vi "ReadPath.vi"(8 "error in (no error)":errorcluster, 11 "AI_Snake in":refnum<class "AI_Snake.lvclass">) -> (0 "error out":errorcluster, 3 "AI_Snake out":refnum<class "AI_Snake.lvclass">)   [LabVIEW 2019, in "RT_Game.lvlib" / "AI_Snake.lvclass"]
uses:
  AI_Snake.lvclass
  C:/Users/FreshBob/Dropbox/VIs/myRIO_GameConsole/RT/RT_Game/Snake/Snake.lvclass
  Engine/Coordinate.ctl
  AI_Snake.lvclass/AI_Snake.ctl
  Snake/Snake.lvclass/Snake.ctl
  Snake/Read Length.vi
  Snake/Write Position (Tiles).vi
  Engine/Engine.lvclass
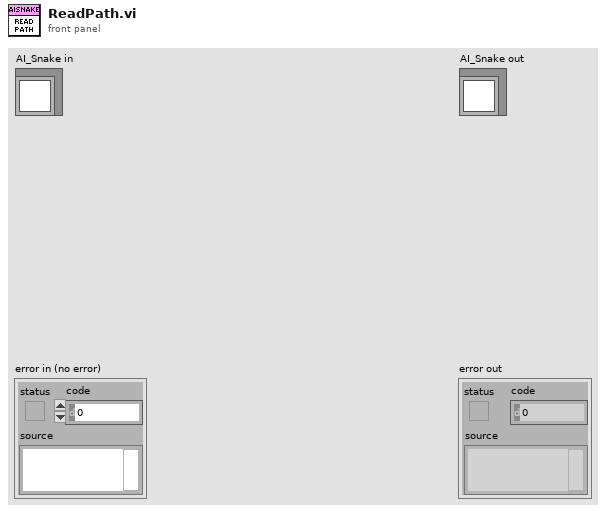
[diagram p1: front panel]
types:
  T1 = typedef "RT_Game.lvlib/Engine.lvclass/Coordinate.ctl" = cluster{"x":dbl, "y":dbl}
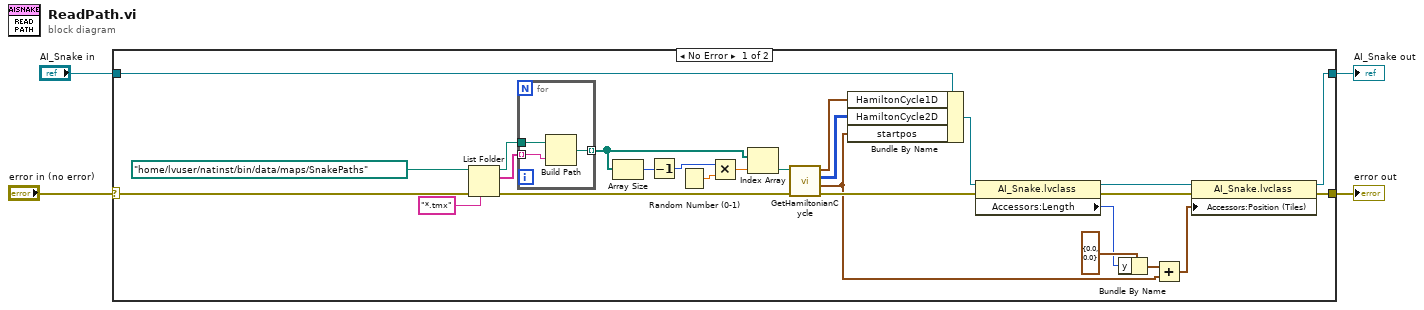
[diagram p0: block diagram]
diagram:
  n1 = case shown="No Error" "error in (no error)" {
    selector: "error in (no error)" -> [w24 w35]
    tunnel: [w23 w35] -> w3
    tunnel: [w21 w34] -> w1
    tunnel: "AI_Snake in" -> [w22 w34]
    frame No Error {
      n2 = List Folder(path=path "/home/lvuser/natinst/bin/data/maps/SnakePaths", pattern="*.tmx", error in=w24) -> (path out=w11:path, filenames=w12:string[], error out=w15:errorcluster)  [unwired: 1 in, 1 out]
      n3 = for {
        tunnel: w12 -> [w33] mode=indexing
        tunnel: w11 -> [w32]
        tunnel: [w31] -> w10 mode=indexing
        n4 = Build Path(base path=w32, name or relative path=w33) -> (appended path=w31:path)
      }
      n5 = Array Size(array=w10) -> (size(s)=w9:i32)
      n6 = Decrement(x=w9) -> (x-1=w7:i32)
      n7 = Random Number (0-1)() -> (number: 0 to 1=w8:dbl)
      n8 = Multiply(x=w7, y=w8) -> (x*y=w6:dbl)
      n9 = Index Array(array=w10, index=w6) -> (element=w5:path)
      n10 = call "GetHamiltonianCycle.vi"("error in (no error)"=w15, "path to tmx-file (created with Tiles2D)"=w5) -> ("error out"=w28:errorcluster, "startpos"=w20:cluster{i32, i32}, "Hamilton2D"=w25:u32[][], "Hamilton1D"=w26:cluster{i32, i32}[])  [unwired: 6 in]
      n11 = Bundle By Name(cluster=w22, "HamiltonCycle1D"=w26, "HamiltonCycle2D"=w25, "startpos"=w20) -> (w27:refnum<class "AI_Snake.lvclass">)
      n12 = property class="AI_Snake.lvclass"(reference=w27, error in=w28) -> (reference out=w29:refnum<class "AI_Snake.lvclass">, error out=w30:errorcluster, "Accessors:Length"=w17:i16)
      n13 = Bundle By Name(cluster=T1 {"x"=0.0, "y"=0.0} ("Position (Tiles)"), "y"=w17) -> (w19:T1)
      n14 = Add(x=w19, y=w20) -> (x+y=w16:T1)
      n15 = property class="AI_Snake.lvclass"(reference=w29, error in=w30, "Accessors:Position (Tiles)"=w16) -> (reference out=w21:refnum<class "AI_Snake.lvclass">, error out=w23:errorcluster)
    }
    frame Error {
    }
  }
  "error out" <- w3
  "AI_Snake out" <- w1
